vi "AutoWait.vi"(7 "Reset?":bool, 11 "Array":dbl[](array[numeric]) format="%0.3f") -> (4 "isFinished":bool)   [LabVIEW 2013]
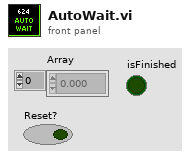
[diagram p1: front panel]
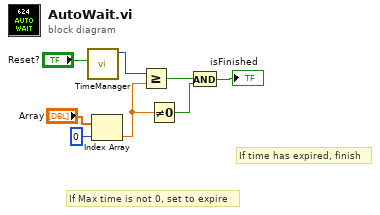
[diagram p0: block diagram]
diagram:
  # "If Max time is not 0, set to expire"
  # "If time has expired, finish"
  n1 = call "TimeManager.vi"("Reset?"="Reset?") -> ("Time Since Reset"=w1:u32)  [unwired: 9 in, 1 out]
  n2 = Index Array(array="Array", index=0) -> (element=w3:dbl)
  n3 = Greater Or Equal?(x=w1, y=w3) -> (x >= y?=w5:bool)
  n4 = Not Equal To 0?(x=w3) -> (x != 0?=w2:bool)
  n5 = And(x=w5, y=w2) -> (x .and. y?=→"isFinished":bool)
